vi "Incrementer.vi"(4 "INC?":bool) -> (1 "count":u32)   [LabVIEW 2011]
doc: "This counter counts from 0....Rollover and then returns to zero\ne.g., If rollover is 2, counter moves as 0,1,2,0,1,2.....\n\n<Latency> = 1 Tick from Reset"
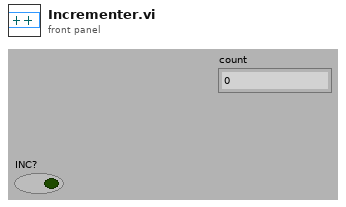
[diagram p1: front panel]
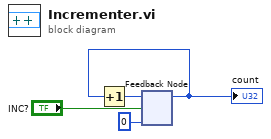
[diagram p0: block diagram]
diagram:
  n1 = feedback #1(u32 0) -> (w1:u32)
  "count" <- w1
  n2 = Increment(x=w1) -> (x+1=w2:u32)
  n3 = feedback-in #1(w2, "INC?") -> ()
